vi "Invert Indices.vi"(4 "Destination Indices":i32[](array[numeric])) -> (7 "Source Indices":i32[](array[numeric]))   [LabVIEW 2020, in "VolatusGUIElements.lvlib"]
uses:
  VolatusGUIElements.lvlib
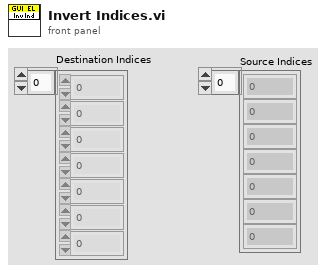
[diagram p1: front panel]
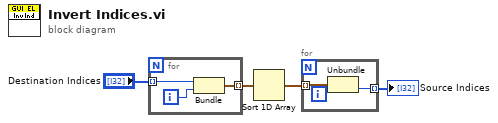
[diagram p0: block diagram]
diagram:
  n1 = for {
    tunnel: "Destination Indices" -> [w7] mode=indexing
    tunnel: [w5] -> w3 mode=indexing
    i -> [w6]
    n2 = Bundle("Numeric"=w7, w6) -> (w5:cluster{"Numeric":i32, i32})  [unwired: 1 in]
  }
  n3 = Sort 1D Array(array=w3) -> (sorted array=w2:cluster{"Numeric":i32, i32}[])
  n4 = for {
    tunnel: w2 -> [w9] mode=indexing
    tunnel: [w8] -> w1 mode=indexing
    n5 = Unbundle(w9) -> (w8:i32)  [unwired: 1 out]
  }
  "Source Indices" <- w1
